vi "PH_PSDBWriter.destructor.vi"(0 "i ref in":refnum<vi>, 5 "error in(no error)":errorcluster) -> (19 "error out":errorcluster)   [LabVIEW 2014, in "PH_PSDBWriter.lvlib"]
doc: "This is the destructor of a class.\n\nLicense Agreement for this software:\n\nCopyright (C)\nGesellschaft für Schwerionenforschung, GSI\nPlanckstr. 1\n64291 Darmstadt\nGermany\n\nContact: D.Beck@gsi.de \n\nThis program is free software; you can redistribute it and/or modify it under the terms of the \nGNU General Public License as published by the Free Software Foundation; either version 2 of \nthe license, or (at your option) any later version.\n\nThis program is distributed in the hope that it will be useful, but WITHOUT ANY WARRANTY; \nwithout even the implied warranty of MERCHANTABILITY or FITNESS FOR A PARTICULAR PURPOSE. See the GNU General License for more details (http://www.gnu.org).\n\nGesellschaft für Schwerionenforschung, GSI\nPlanckstr. 1, 64291 Darmstadt, Germany\nFor all questions and ideas contact: M.Richter@gsi.de, H.Brand@gsi.de or D.Beck@gsi.de.\nLast update: 16-JUN-2004"
uses:
  PH_PSDBWriter.lvlib
  PH_Class/PH_Class.lvlib
  lib.lib/DimLVEvent/LVDimInterface/LVDimInterface.lvlib
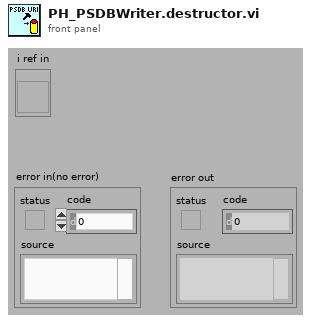
[diagram p1: front panel]
types:
  T1 = typedef "PH_PSDBWriter.lvlib/PH_PSDBWriter.i attribute.ctl" = cluster{"PSDB Status Service ID":i32, "Instance ID":i32, "Shot #":i32, "Subsystem":T2, "Data Status":T3, "Ref PSDB Status":refnum<vi>, "PSDB Error Code":i32, "PSDB Dataset":T4, "PSDB Thread":cluster{"Ref":refnum<vi>, "Q-Ref":refnum<queue>}, "PSDB Credentials":T12}
  T2 = typedef "PH_PSDBWriter.lvlib/PH_PSDBWriter.PHELIX-Subsystems.ctl" = i32
  T3 = typedef "PH_PSDBWriter.lvlib/PH_PSDBWriter.Data Status.ctl" = i16
  T4 = typedef "PH_PSDBWriter.lvlib/PH_PSDBWriter.PSDB Dataset.ctl" = cluster{"Version":i32, "2D data Input":T5[], "Boolean Input":T7[], "Image Input":T8[], "Numeric Input":T10[], "String Input":T11[]}
  T5 = typedef "PH_PSDBWriter.lvlib/PH_PSDBWriter.2D dataset.ctl" = cluster{"name":string, "data":dbl[][], "axis description":T6}
  T6 = typedef "PSDB.lvlib/PSDB_AxisDescription.ctl" = cluster{"x axis label":string, "y axis label":string, "x axis unit":string, "y axis unit":string}
  T7 = typedef "PH_PSDBWriter.lvlib/PH_PSDBWriter.Boolean dataset.ctl" = cluster{"name":string, "data":bool, "unit":string}
  T8 = typedef "PH_PSDBWriter.lvlib/PH_PSDBWriter.Image dataset.ctl" = cluster{"name":string, "data":T9, "unit":string}
  T9 = typedef "IMAQ Image.ctl" = refnum<image>
  T10 = typedef "PH_PSDBWriter.lvlib/PH_PSDBWriter.Numeric dataset.ctl" = cluster{"name":string, "data":dbl, "unit":string}
  T11 = typedef "PH_PSDBWriter.lvlib/PH_PSDBWriter.String dataset.ctl" = cluster{"name":string, "data":string, "unit":string}
  T12 = typedef "PH_Common.lvlib/PH_Connection.PSDB Credentials.ctl" = cluster{"PW":string, "ID":string, "DS":string}
  T13 = enum16{"SetAttribute", "GetAttribute", "CreateAttribute", "DestroyAttribute", "DestroyAllAtributes"}
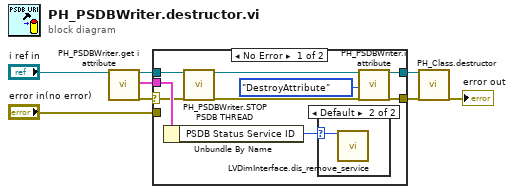
[diagram p0: block diagram]
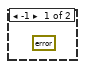
[diagram p2: hidden frame]
diagram:
  n1 = call "PH_PSDBWriter.get i attribute.vi"("i ref in"="i ref in") -> ("i ref out"=w6:refnum<vi>, "i attribute"=w2:T1, "error out"=w8:errorcluster)  [unwired: 16 in]
  n2 = case shown="No Error" w8 {
    selector: w8 -> [w15 _]
    tunnel: [w10 w19] -> w4
    tunnel: w6 -> [w16 w20]
    tunnel: [w12 w20] -> w3
    tunnel: w2 -> [w17 _]
    tunnel: "error in(no error)" -> [_ w19]
    frame No Error {
      n3 = Unbundle By Name(w17) -> ("PSDB Status Service ID"=w14:i32)
      n4 = call "PH_PSDBWriter.STOP PSDB THREAD.vi"("VI in"=w16, "error in (no error)"=w15) -> ("VI out"=w13:refnum<vi>, "error out"=w11:errorcluster)  [unwired: 16 in]
      n5 = case shown="Default" w14 {
        selector: w14 -> [_ w18]
        frame -1 {
          (unwired) errorcluster {"status"=FALSE, "code"=0, "source"=""} ("error out")
        }
        frame Default {
          n6 = call "LVDimInterface.dis_remove_service.vi"("my_serviceID"=w18) -> ()  [unwired: 18 in, 1 out]
        }
      }
      n7 = call "PH_PSDBWriter.i attribute.vi"("VI Refnum"=w13, "Action"=T13."DestroyAttribute", "error in (no error)"=w11) -> ("VI Refnum out"=w12:refnum<vi>, "error out"=w10:errorcluster)  [unwired: 14 in, 1 out]
    }
    frame Error {
    }
  }
  n8 = call "PH_Class.destructor.vi"("i ref in"=w3, "error in(no error)"=w4) -> ("error out"=→"error out":errorcluster)  [unwired: 17 in]
